vi "video_camera_test.vi"() -> ()   [LabVIEW 2011]
panel:
  in  "Stop (F) 2":bool caption="Stop (F)"
  out "Image Out 2":T1(plugin-control)
  in  "stop":bool
  in  "Stop (F)":bool
  out "Image Out":T1(plugin-control)
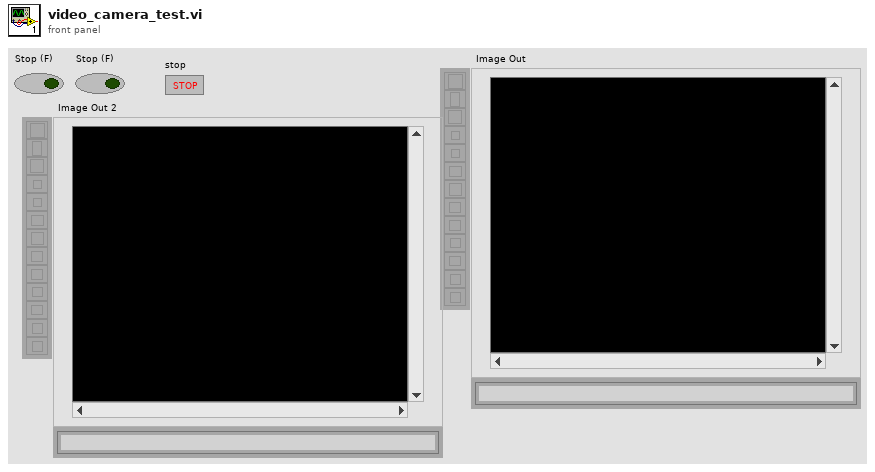
[diagram p1: front panel]
types:
  T1 = typedef "IMAQ Image.ctl" = refnum<image>
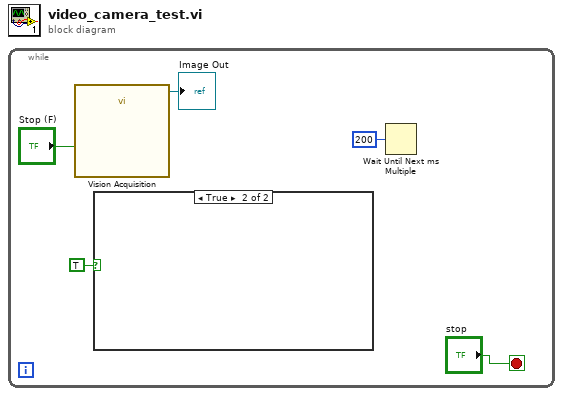
[diagram p0: block diagram]
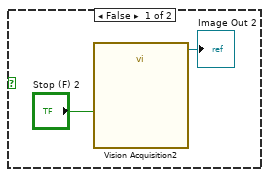
[diagram p2: hidden frame]
diagram:
  n1 = while {
    stop <- "stop" stop-if-true
    n2 = call "Vision Acquisition"("Stop (F)"="Stop (F)") -> ("Image Out"=→"Image Out":T1)  [unwired: 24 in, 2 out]
    n3 = case shown="True" TRUE {
      frame False {
        n4 = call "Vision Acquisition2"("Stop (F)"="Stop (F) 2") -> ("Image Out"=→"Image Out 2":T1)  [unwired: 24 in, 2 out]
      }
      frame True {
      }
    }
    n5 = Wait Until Next ms Multiple(millisecond multiple=u32 200) -> ()  [unwired: 1 out]
  }
